vi "Unregister Data Logging Events.vi"(8 "error in (no error)":errorcluster, 11 "Registered Data Logging Event Refnum":T1) -> (0 "error out":errorcluster)   [LabVIEW 2020, in "NI_VS Data Logging API.lvlib"]
doc: "Unregisters for data logging events from the VeriStand Gateway."
uses:
  <vilib>/NI VeriStand/Execution/DataLogging/NI_VS Data Logging API.lvlib
  <vilib>/NI VeriStand/Execution/DataLogging/Registered Data Logging Event Refnum.ctl
  <vilib>/NI VeriStand/Execution/DataLogging/Data Logging User Event Refs.ctl
  <vilib>/NI VeriStand/Execution/DataLogging/Data Logging Session Error Event Data.ctl
  <vilib>/NI VeriStand/Execution/DataLogging/Data Logging Session Start Event Data.ctl
  <vilib>/NI VeriStand/Execution/DataLogging/Data Logging Session State Change Event Data.ctl
  <vilib>/NI VeriStand/Execution/DataLogging/Data Logging Session State.ctl
  <vilib>/NI VeriStand/Execution/DataLogging/Data Logging Session Stop Event Data.ctl
  <vilib>/NI VeriStand/Execution/DataLogging/Log File Closed Event Data.ctl
  <vilib>/NI VeriStand/Execution/DataLogging/Log File Opened Event Data.ctl
  <vilib>/NI VeriStand/Execution/DataLogging/New Log Files Complete Event Data.ctl
  <vilib>/NI VeriStand/Execution/DataLogging/Data Logging Event Registration Refnum.ctl
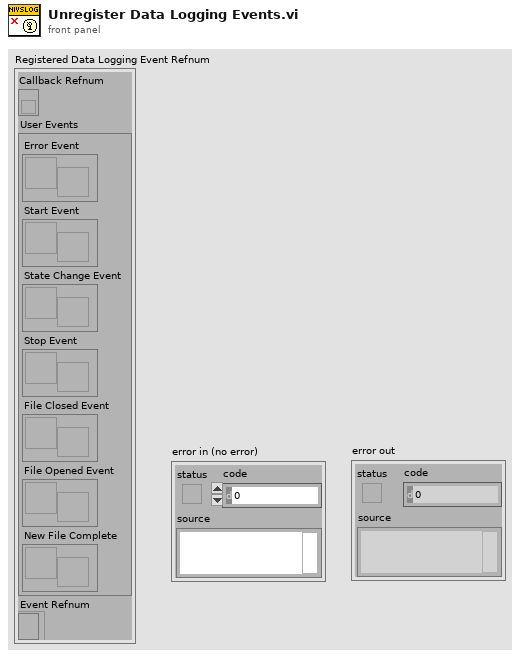
[diagram p1: front panel]
types:
  T1 = typedef "NI_VS Data Logging API.lvlib/Registered Data Logging Event Refnum.ctl" = cluster{"Callback Refnum":refnum<k27>, "User Events":T2, "Event Refnum":T3}
  T2 = typedef "NI_VS Data Logging API.lvlib/Data Logging User Event Refs.ctl" = cluster{"Error Event":refnum<user-event>, "Start Event":refnum<user-event>, "State Change Event":refnum<user-event>, "Stop Event":refnum<user-event>, "File Closed Event":refnum<user-event>, "File Opened Event":refnum<user-event>, "New File Complete":refnum<user-event>}
  T3 = typedef "NI_VS Data Logging API.lvlib/Data Logging Event Registration Refnum.ctl" = refnum<event-registration>
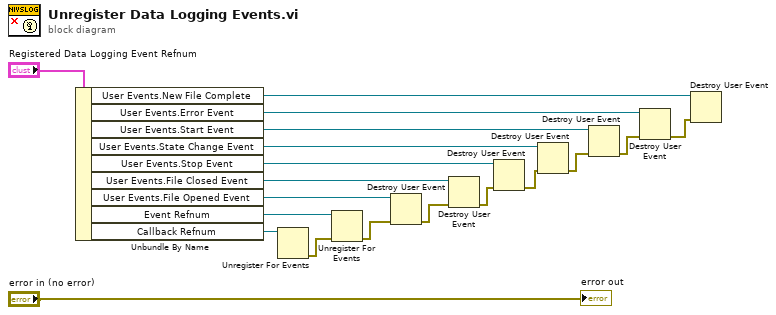
[diagram p0: block diagram]
diagram:
  n1 = Unbundle By Name("Registered Data Logging Event Refnum") -> ("User Events.New File Complete"=w2:refnum<user-event>, "User Events.Error Event"=w5:refnum<user-event>, "User Events.Start Event"=w7:refnum<user-event>, "User Events.State Change Event"=w9:refnum<user-event>, "User Events.Stop Event"=w11:refnum<user-event>, "User Events.File Closed Event"=w13:refnum<user-event>, "User Events.File Opened Event"=w15:refnum<user-event>, "Event Refnum"=w16:T3, "Callback Refnum"=w18:refnum<k27>)
  n2 = Unregister For Events(event registration refnum=w18) -> (error out=w17:errorcluster)  [unwired: 1 in]
  n3 = Unregister For Events(event registration refnum=w16, error in=w17) -> (error out=w14:errorcluster)
  n4 = Destroy User Event(user event=w15, error in=w14) -> (error out=w12:errorcluster)
  n5 = Destroy User Event(user event=w13, error in=w12) -> (error out=w10:errorcluster)
  n6 = Destroy User Event(user event=w11, error in=w10) -> (error out=w8:errorcluster)
  n7 = Destroy User Event(user event=w9, error in=w8) -> (error out=w6:errorcluster)
  n8 = Destroy User Event(user event=w7, error in=w6) -> (error out=w4:errorcluster)
  n9 = Destroy User Event(user event=w5, error in=w4) -> (error out=w1:errorcluster)
  n10 = Destroy User Event(user event=w2, error in=w1) -> ()  [unwired: 1 out]
  "error out" <- "error in (no error)"
